vi "onCreate.vi"(8 "error in (no error)":errorcluster, 11 "Pump.Simulated":refnum<class "Pump.Simulated.lvclass">) -> (0 "error out":errorcluster, 3 "Pump.Simulated out":refnum<class "Pump.Simulated.lvclass">)   [LabVIEW 2014, in "Pump.Simulated.lvclass"]
doc: "JKI State Machine Objects (SMO) 1.4.0.57\nJKI - JKI\nCopyright (c) 2018, JKI"
uses:
  Pump.Simulated.lvclass
  Pump.Simulated.lvclass/Pump.Simulated.ctl
  Pump class/Pump.lvclass
panel:
  # "For instructions on how to use the JKI State Machine Objects, examples and video tutorials, visit:\nhttp://jki.net/state-machine-objects/\n\nJKI State Machine Objects™\nhttp://jki.net/state-machine-objects/\nCopyright (C) 2005-2015, JKI <info@jki.net>\nALL RIGHTS RESERVED"
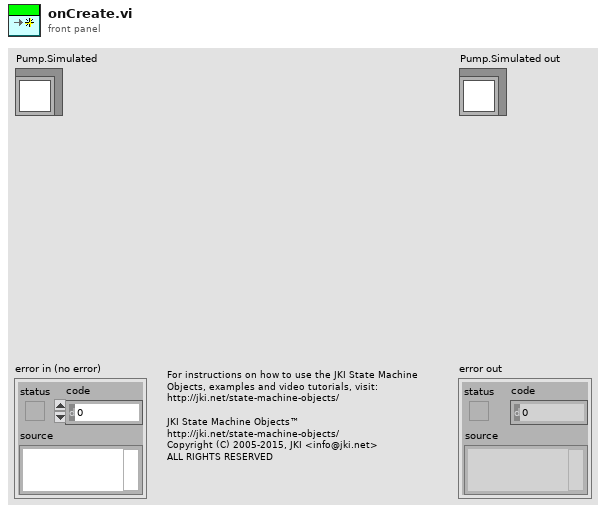
[diagram p1: front panel]
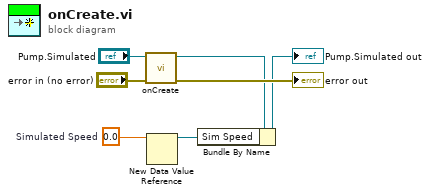
[diagram p0: block diagram]
diagram:
  w4 = 0.0  # Simulated Speed
  n1 = call-parent "onCreate.vi"("error in (no error)"="error in (no error)", "Pump"="Pump.Simulated") -> ("error out"=→"error out":errorcluster, "Pump out"=w2:refnum<class "Pump.Simulated.lvclass">)  [unwired: 8 in]
  n2 = New Data Value Reference(data value=w4) -> (data value reference=w3:refnum<data-value>)  [unwired: 1 in, 1 out]
  n3 = Bundle By Name(cluster=w2, "Sim Speed"=w3) -> (→"Pump.Simulated out":refnum<class "Pump.Simulated.lvclass">)
